vi "Chip to String.vi"(8 "error in (no error)":errorcluster, 11 "MPLab in":refnum<class "MPLab.lvclass">) -> (0 "error out":errorcluster, 3 "MPLab out":refnum<class "MPLab.lvclass">)   [LabVIEW 2018, in "MPLab.lvlib" / "MPLab.lvclass"]
uses:
  MPLab.lvclass
  MPLab.lvclass/MPLab.ctl
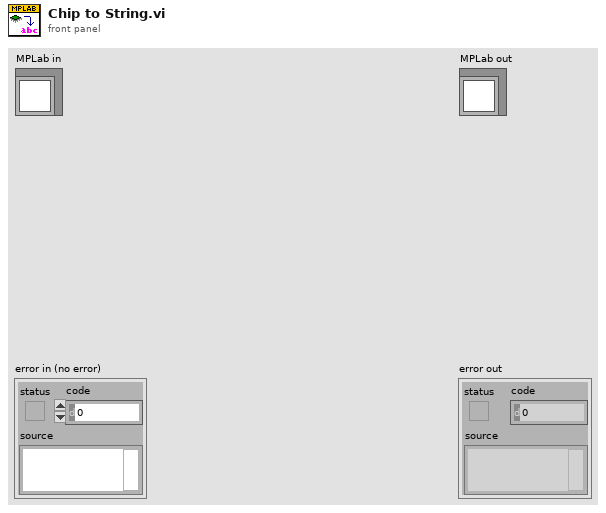
[diagram p1: front panel]
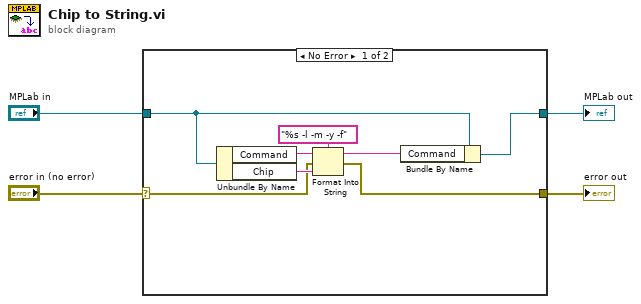
[diagram p0: block diagram]
diagram:
  n1 = case shown="No Error" "error in (no error)" {
    selector: "error in (no error)" -> [w5 w13]
    tunnel: "MPLab in" -> [w9 w14]
    tunnel: [w8 w14] -> w3
    tunnel: [w6 w13] -> w2
    frame No Error {
      n2 = Unbundle By Name(w9) -> ("Command"=w12:string, "Chip"=w11:string)
      n3 = Format Into String(format string="%s -l -m -y -f", initial string=w12, error in=w5, w11) -> (resulting string=w7:string, error out=w6:errorcluster)
      n4 = Bundle By Name(cluster=w9, "Command"=w7) -> (w8:refnum<class "MPLab.lvclass">)
    }
    frame Error {
    }
  }
  "error out" <- w2
  "MPLab out" <- w3
